vi "case_initialize.vi"(7 "Main VI reference":refnum<vi>, 8 "error in (no error)":errorcluster, 9 "message cluster":T2, 10 "Config refnum in":T1, 11 "VISA resource name in":refnum<visa-resource-name>) -> (0 "error out":errorcluster, 1 "initialized":bool, 2 "Config refnum out":T1, 3 "VISA resource name out":refnum<visa-resource-name>)   [LabVIEW 2020]
uses:
  controls/message cluster.ctl
  <vilib>/Utility/config.llb/Config Data RefNum.ctl
  5944bac6-5ddb-4f5b-96e6-576bfc250b21.vi
  a0d43237-6b6b-4176-8c88-8eae8e8013ac.vi
  <vilib>/Utility/config.llb/Read Key (String).vi
  <vilib>/Utility/config.llb/NI_LVConfig.lvlib
  <instrlib>/Marlin Instrument Driver/Marlin Instrument Driver.lvlib
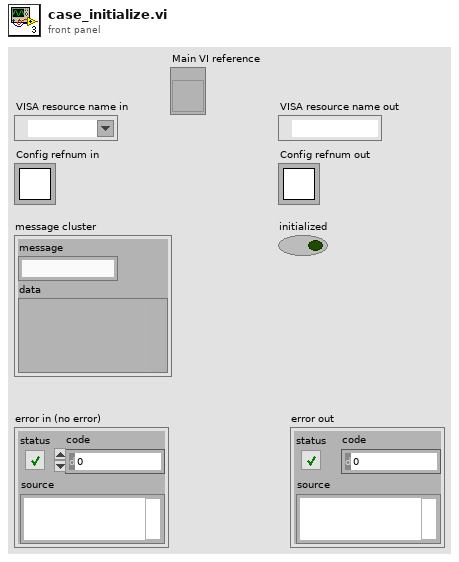
[diagram p1: front panel]
types:
  T1 = typedef "NI_LVConfig.lvlib/Config Data RefNum.ctl" = refnum<k1>
  T2 = typedef "message cluster.ctl" = cluster{"message":string, "data":variant}
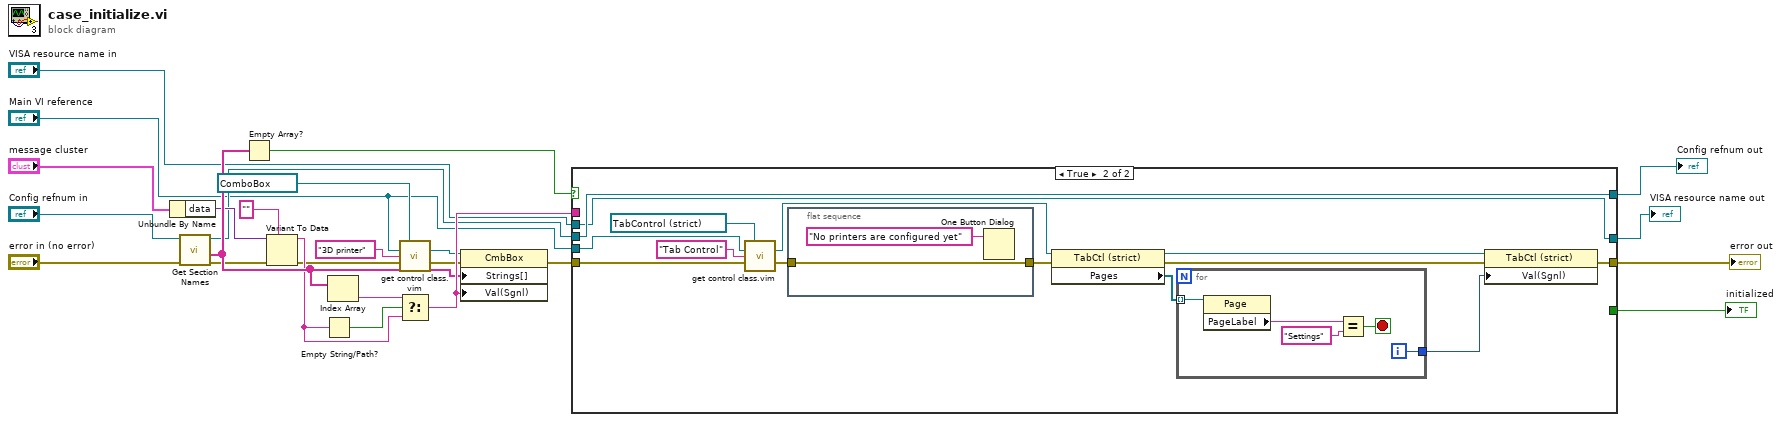
[diagram p0: block diagram]
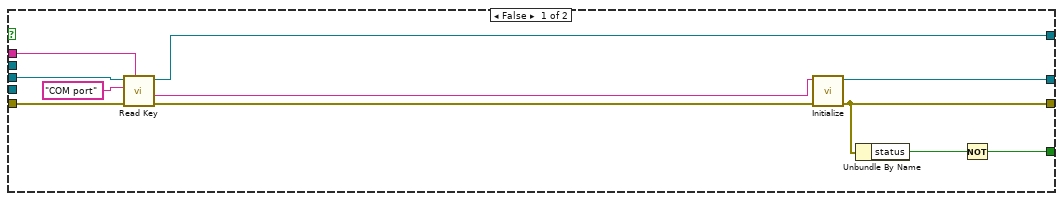
[diagram p2: hidden frame]
diagram:
  n1 = Unbundle By Name("message cluster") -> ("data"=w17:variant)
  n2 = call <vilib>:"Get Section Names.vi"("error in (no error)"="error in (no error)", "refnum"="Config refnum in") -> ("error out"=w2:errorcluster, "section names"=w23:string[], "refnum out"=w9:T1)  [unwired: 7 in]
  n3 = Empty Array?(array=w23) -> (empty?=w8:bool)
  n4 = Variant To Data(error in=w2, type="", Variant=w17) -> (data=w21:string, error out=w1:errorcluster)
  n5 = Empty String/Path?(string/path=w21) -> (empty?=w20:bool)
  n6 = Index Array(array=w23) -> (element=w24:string)  [unwired: 1 in]
  n7 = call "get control class.vim"("Control class"=refnum<vi> refnum, "Main VI reference"="Main VI reference", "Label"="3D printer", "error in (no error)"=w1) -> ("Control out"=w6:refnum<vi>, "error out"=w4:errorcluster)  [unwired: 10 in]
  n8 = Select(t=w24, s=w20, f=w21) -> (s? t:f=w25:string)
  n9 = property on="Property Node" class="CmbBox"(reference=w6, error in=w4, "Strings[]"=w23, "Val(Sgnl)"=w25) -> (error out=w22:errorcluster)  [unwired: 1 out]
  n10 = case shown="True" w8 {
    tunnel: w9 -> [w36 w50]
    tunnel: [w33 w46] -> w10
    tunnel: [w29 w47] -> w11
    tunnel: w22 -> [w31 w40]
    tunnel: [w30 w50] -> w12
    tunnel: [w27 _] -> w13
    tunnel: "VISA resource name in" -> [_ w46]
    tunnel: w25 -> [w26 _]
    tunnel: "Main VI reference" -> [_ w42]
    frame False {
      n11 = call-poly <vilib>:"Read Key.vi"("section"=w26, "error in (no error)"=w31, "key"="COM port", "refnum"=w36) -> ("error out"=w32:errorcluster, "value"=w34:string, "refnum out"=w30:T1)  [unwired: 4 in, 1 out]
      n12 = call <instrlib>:"Initialize.vi"("error in (no error)"=w32, "VISA resource name"=w34) -> ("error out"=w29:errorcluster, "VISA resource name out"=w33:refnum<visa-resource-name>)  [unwired: 8 in]
      n13 = Unbundle By Name(w29) -> ("status"=w28:bool)
      n14 = Not(x=w28) -> (.not. x?=w27:bool)
    }
    frame True {
      n15 = call "get control class.vim"("Control class"=refnum<vi> refnum ("Tab Control"), "Main VI reference"=w42, "Label"="Tab Control", "error in (no error)"=w40) -> ("Control out"=w38:refnum<vi>, "error out"=w39:errorcluster)  [unwired: 10 in]
      n16 = flat-sequence {
        tunnel: [w56] -> w49
        tunnel: w39 -> [w56]
        frame #0 {
          n17 = One Button Dialog(message="No printers are configured yet") -> ()  [unwired: 1 in, 1 out]
        }
      }
      n18 = property on="Property Node" class="TabCtl (strict)"(reference=w38, error in=w49) -> (reference out=w43:refnum<vi>, error out=w48:errorcluster, "Pages"=w45:refnum<vi>[])
      n19 = for {
        tunnel: w45 -> [w55] mode=indexing
        tunnel: [w51] -> w44
        i -> [w51]
        stop <- w52 stop-if-true
        n20 = property class="Page"(reference=w55) -> ("PageLabel"=w54:string)  [unwired: 1 in, 2 out]
        n21 = Equal?(x=w54, y="Settings") -> (x = y?=w52:bool)
      }
      n22 = property on="Property Node" class="TabCtl (strict)"(reference=w43, error in=w48, "Val(Sgnl)"=w44) -> (error out=w47:errorcluster)  [unwired: 1 out]
    }
  }
  "initialized" <- w13
  "Config refnum out" <- w12
  "error out" <- w11
  "VISA resource name out" <- w10
